vi "SafeMoving.vi"() -> ()   [LabVIEW 2016]
uses:
  Control/SafeControl.ctl
  Control/SafeMoveControl.ctl
  Other Models/2010/Motion/EnableSingle.vi
  Other Models/2010/Motion/DisableSingle.vi
  C:/Users/TTUHEP/Documents/LabVIEW/Other Models/2010/Bin/Aerotech.A3200.dll
  Other Models/2010/Bin/Aerotech.A3200.dll
panel:
  out "Velocity U":dbl
  out "Position U":dbl
  out "Program Position U":dbl
  in  "HOME U":bool
  out "U":string
  out "U":bool
  in  "Enable U":bool
  in  "Axis":enum16{"Z", "Y", "X"}(ring)
  in  "Axis2":string
  in  "Stop3":bool caption="Pause/resume"
  in  "Stop1":bool caption="Pause/resume"
  in  "Move down 2":bool caption="Move"
  in  "Move up 2":bool caption="Move"
  in  "Tab Control":enum32{"Free", "Steps", "Total"}(tab)
  in  "Speed(µm)":dbl=500.0
  in  "Dis/Step(µm)":dbl=5.0
  in  "Step":i32=1
  in  "Dis/step(µm)":dbl=5.0
  in  "Speed(µm/s)":dbl=500.0
  in  "Speed(µm/s) 2":dbl=500.0
  in  "Total Distance(µm)":dbl=5.0
  in  "Dis/step(µm) 2":dbl=1.0
  in  "Pause":bool caption="Pause/resume"
  in  "Resume":bool caption="Pause/resume"
  in  "Move down":bool caption="Move"
  in  "Move up":bool caption="Move"
  out "Boolean":bool
  out "Velocity Z":dbl
  out "Position Z":dbl
  out "Program Position Z":dbl
  out "Velocity Y":dbl
  out "Position Y":dbl
  out "Program Position Y":dbl
  out "Program Position X":dbl
  out "Position X":dbl
  out "Velocity X":dbl format="%#.5g"
  in  "Excute":bool
  in  "HOME Z":bool
  in  "HOME Y":bool
  in  "HOME X":bool
  out "Y":string
  out "Z":string
  out "X":string caption="Status"
  in  "Exit":bool
  out "Z":bool
  out "Y":bool
  out "X":bool
  in  "Enable Z":bool
  in  "Enable Y":bool
  in  "Enable X":bool
  in  "Command":string
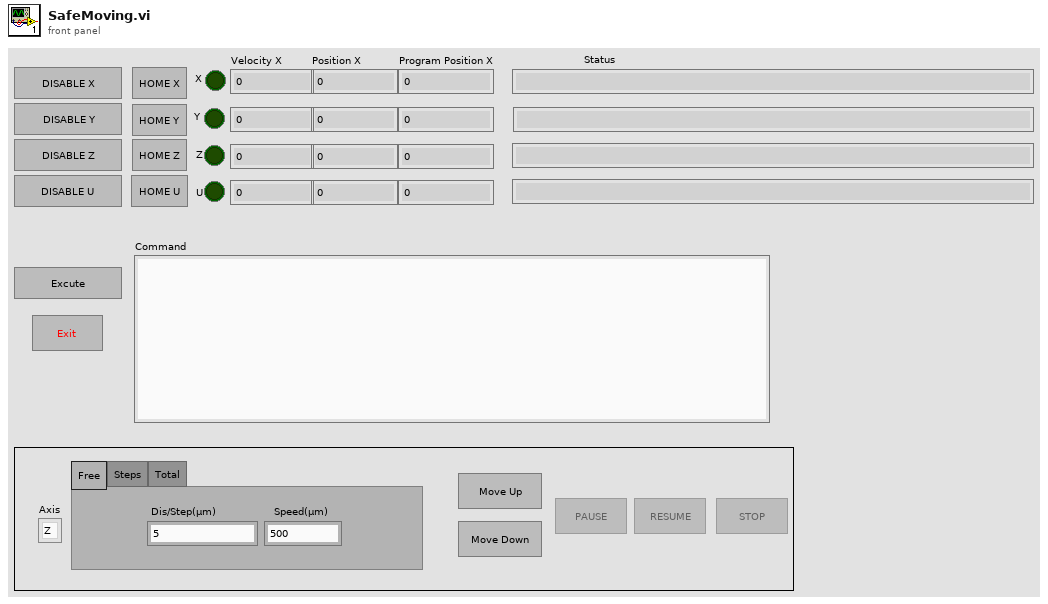
[diagram p1: front panel]
types:
  T1 = typedef "SafeMoveControl.ctl" = enum16{"Idle", "Pause", "Run2", "Run1"}
  T2 = typedef "SafeControl.ctl" = enum16{"Idle", "Abort", "Initialize", "BeforeExcute"}
  T3 = cluster{"X":bool, "Y":bool, "Z":bool, "X":string, "Y":string, "Z":string, "U":bool, "U":string}
  T4 = enum8{"Enabled", "Disabled", "Disabled and Grayed Out"}
  T5 = typedef "ControllerDiagPacket.ctl" = cluster{"Number of Diag Packets":i32, "Axes":T6[], "error":errorcluster}
  T6 = typedef "AxisDiagPacket.ctl" = cluster{"Axis Name":string, "Analog Input 0":dbl, "Analog Input 1":dbl, "Axis Fault (num)":i32, "Axis Fault (str)":string, "Axis Fault (bits)":cluster{"AmplifierFault":bool, "AmplifierTemperatureFault":bool, "CcwEndOfTravelLimitFault":bool, "CcwSoftwareLimitFault":bool, "CommunicationLostFault":bool, "CwEndOfTravelLimitFault":bool, "CwSoftwareLimitFault":bool, "EmergencyStopFault":bool, "EncoderFault":bool, "ExternalFault":bool, "FeedbackScalingFault":bool, "GantryMisalignFault ":bool, "HallSensorFault":bool, "InPositionTimeoutFault":bool, "InternalFault":bool, "MarkerSearchFault":bool, "MaxVelocityCommandFault":bool, "MissedInterruptFault":bool, "MotorTemperatureFault":bool, "None":bool, "OverCurrentFault":bool, "PositionErrorFault":bool, "PositionFeedbackFault":bool, "PowerSupplyFault":bool, "ProbeInputFault":bool, "SafeZoneFault":bool, "VelocityErrorFault":bool, "VelocityFeedbackFault":bool, "VoltageClampFault":bool}, "Axis Status (num)":i32, "Axis Status (str)":string, "Axis Status (bits)":cluster{"BacklashActive":bool, "CalibrationEnabled1D":bool, "CalibrationEnabled2D":bool, "CommandValid":bool, "DriveAbortPending":bool, "DrivePending":bool, "Enabling":bool, "GainMappingEnabled":bool, "GantryAligned":bool, "GantryRealigning":bool, "Homed":bool, "Homing":bool, "IFOVEnabled":bool, "JogGenerating":bool, "Jogging":bool, "JoystickControl":bool, "MasterSlaveControl":bool, "MotionBlocked":bool, "MotionClamped":bool, "MoveDone":bool, "None":bool, "NotVirtual":bool, "Profiling":bool, "Stability0":bool, "Stability1":bool, "TrajectoryFiltering":bool, "WaitDone":bool}, "Current Command":sgl, "Current Error":sgl, "Current Feedback":sgl, "Digital Inputs":i32, "Digital Outputs":i32, "Drive Status":i32, "Drive Status (str)":string, "Drive Status (bits)":cluster{"AccelerationPhase":bool, "AutofocusActive":bool, "BrakeOutput":bool, "CcwEndOfTravelLimitInput":bool, "CosineEncoderError":bool, "CurrentClamp":bool, "CwEndOfTravelLimitInput":bool, "DecelerationPhase":bool, "DualLoopActive":bool, "EmergencyStopInput":bool, "Enabled":bool, "EncoderClipping":bool, "GalvoCalibrationEnabled":bool, "GalvoPowerCorrection":bool, "HallAInput":bool, "HallBInput":bool, "HallCInput":bool, "HighResolutionMode":bool, "HomeLimitInput":bool, "InPosition":bool, "InPosition2":bool, "MarkerInput":bool, "MarkerLatch":bool, "MoveActive":bool, "NoMotorSupply":bool, "None":bool, "PowerLimiting":bool, "ProgrammingFlash":bool, "ProgrammingMXH":bool, "PSOHaltLatch":bool, "ServoControl":bool, "SineEncoderError":bool}, "Position Feedback Auxiliary":dbl, "Position Command":dbl, "Position Error":dbl, "Position Feedback":dbl, "Program Position Command":dbl, "Program Position Error":dbl, "Program Position Feedback":dbl, "Velocity Command":dbl, "Velocity Error":dbl, "Velocity Feedback":dbl}
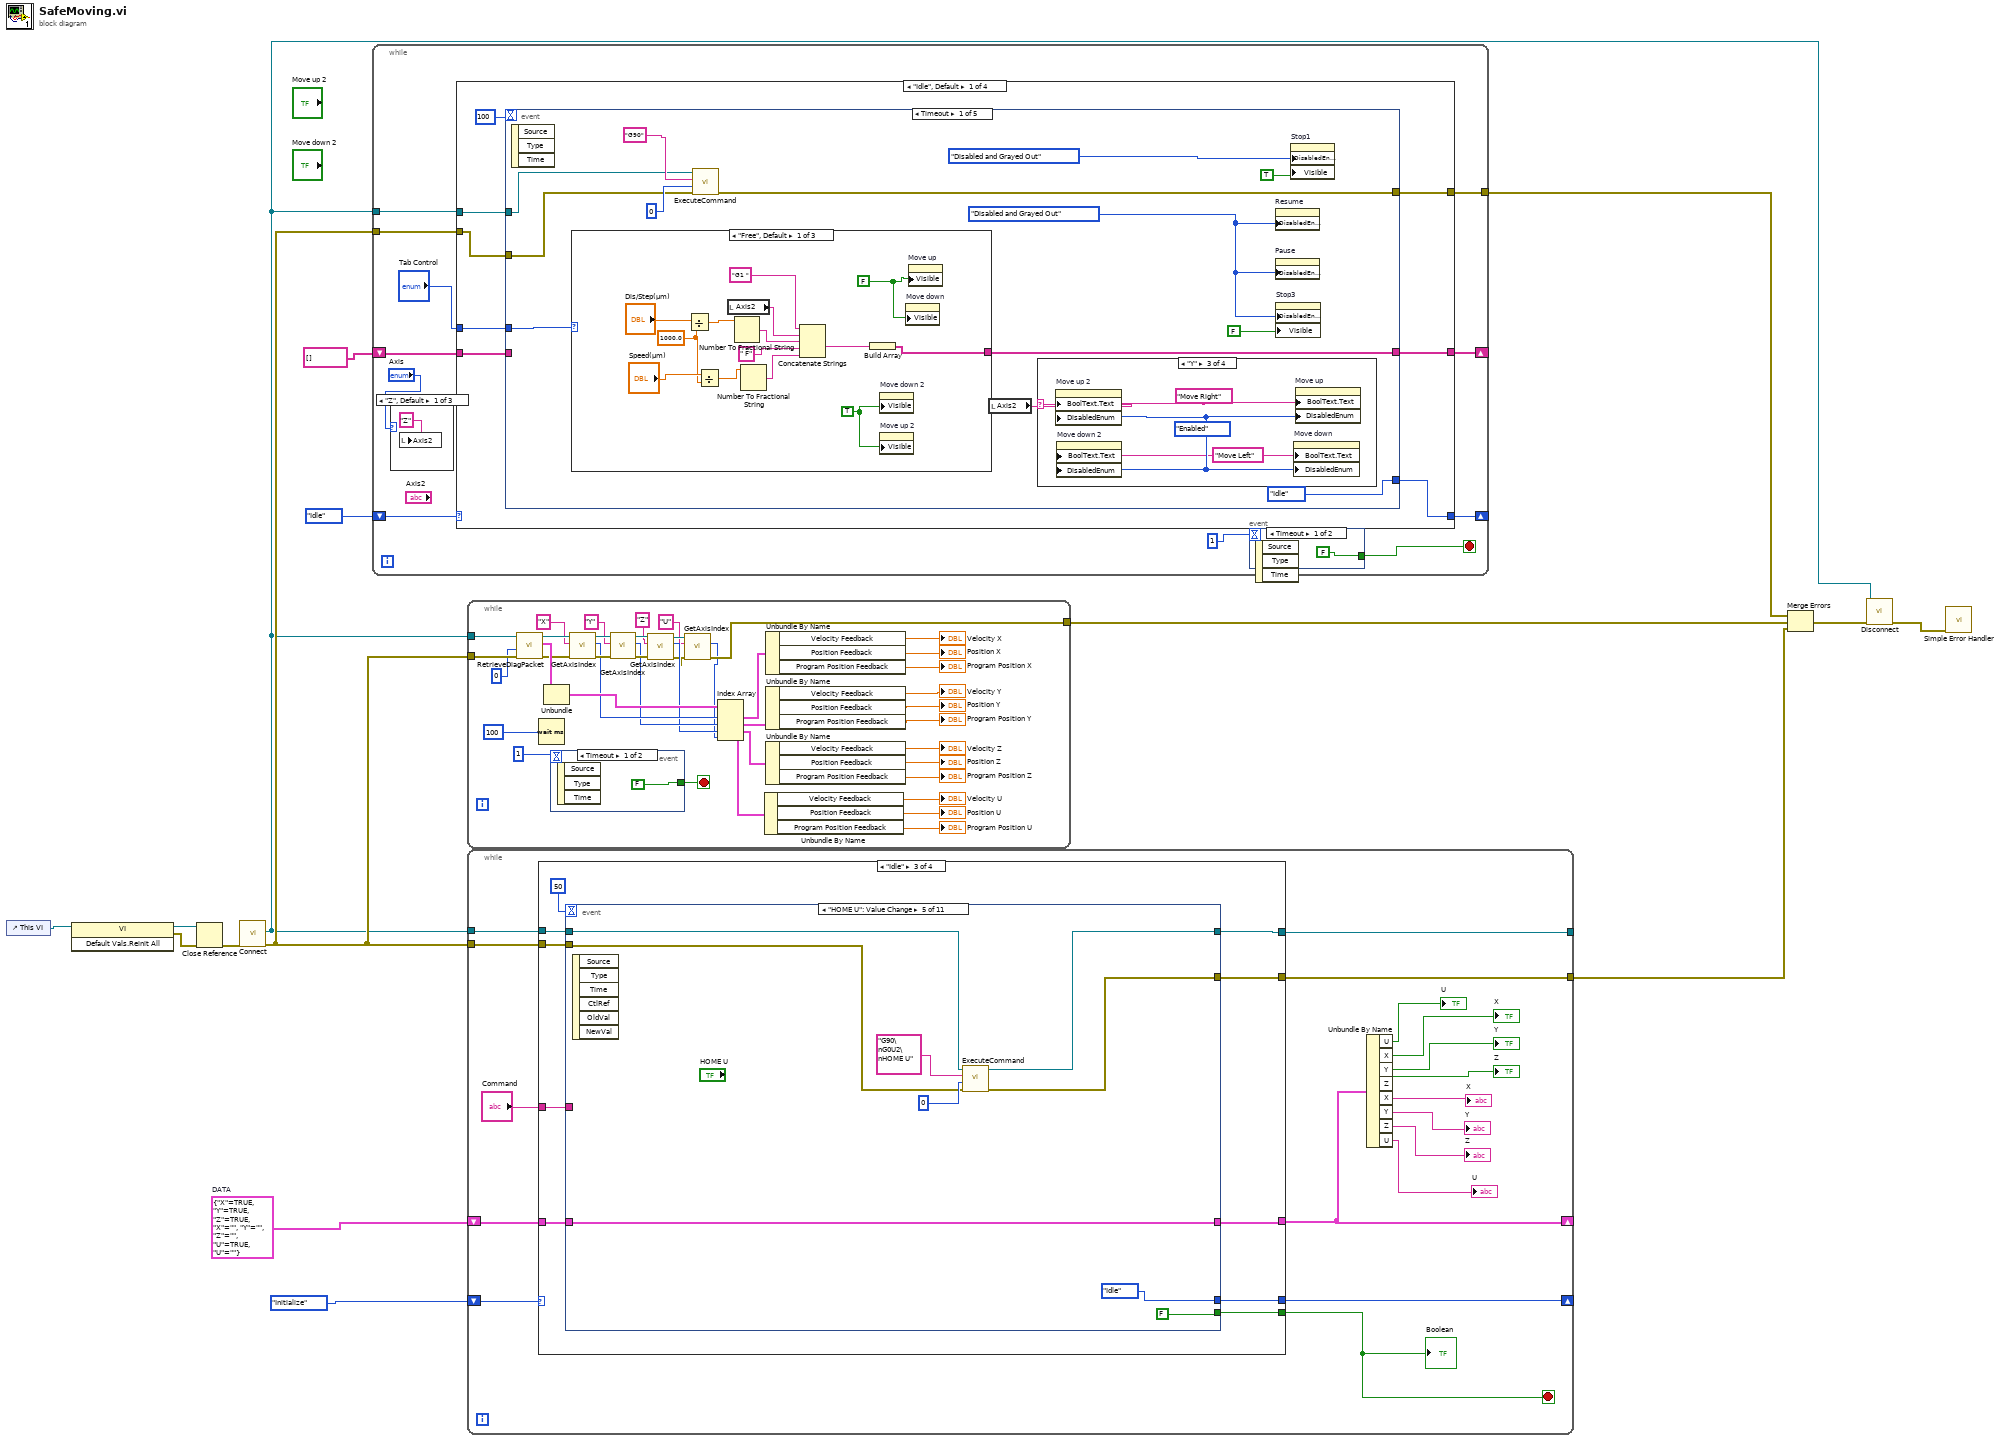
[diagram p0: block diagram]
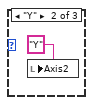
[diagram p2: hidden frame]
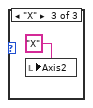
[diagram p3: hidden frame]
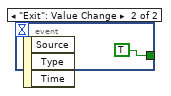
[diagram p4: hidden frame]
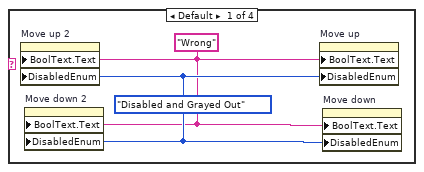
[diagram p5: hidden frame]
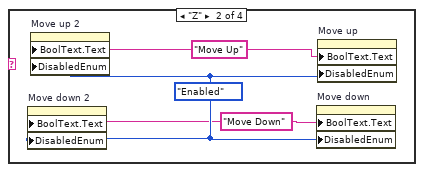
[diagram p6: hidden frame]
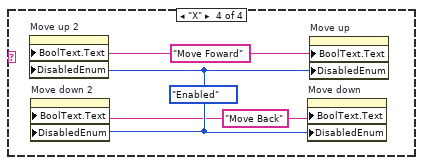
[diagram p7: hidden frame]
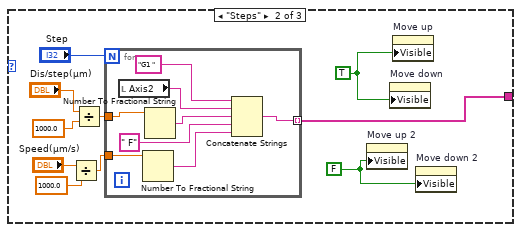
[diagram p8: hidden frame]
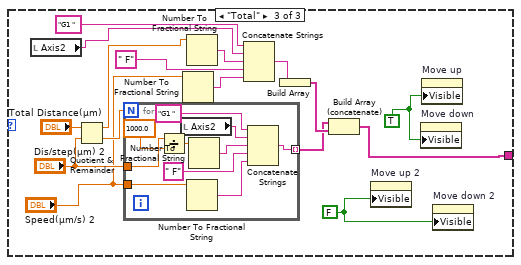
[diagram p9: hidden frame]
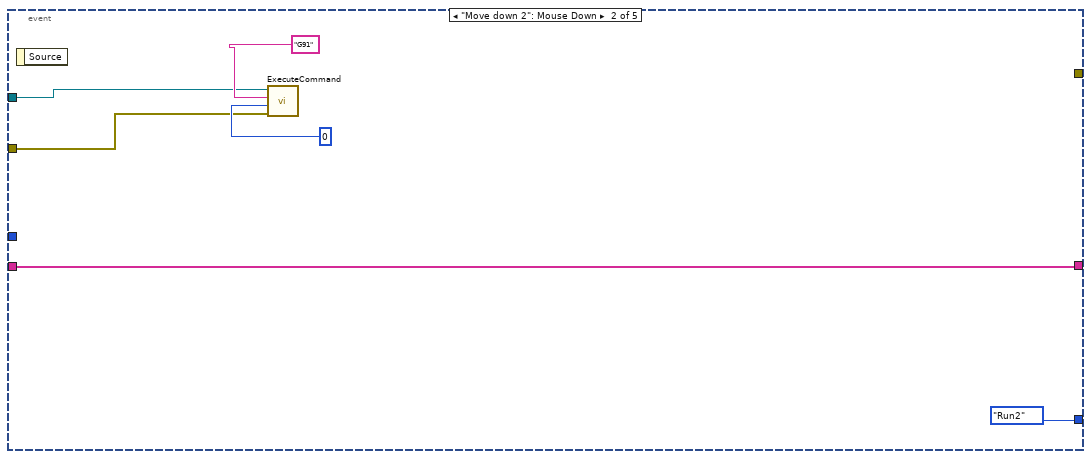
[diagram p10: hidden frame]
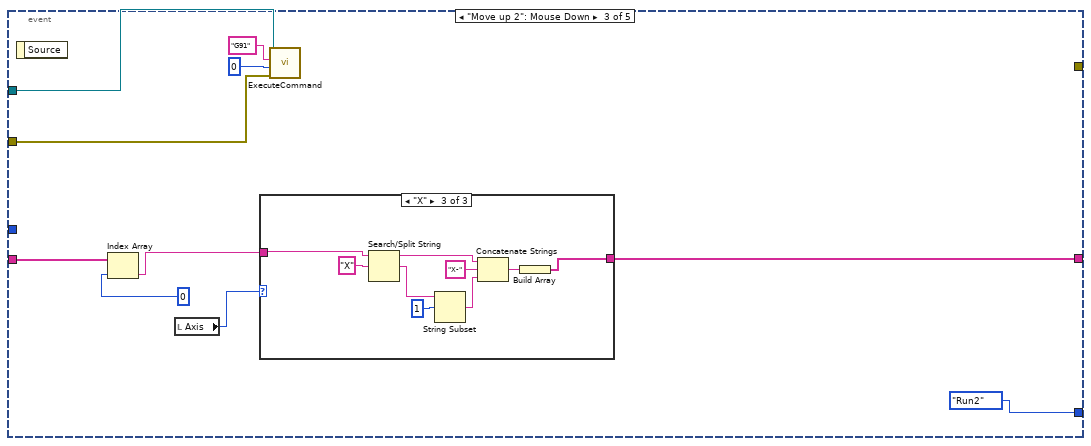
[diagram p11: hidden frame]
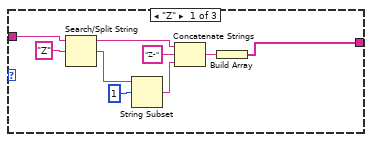
[diagram p12: hidden frame]
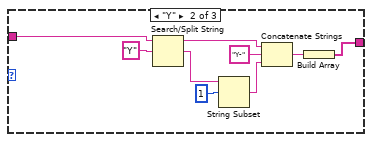
[diagram p13: hidden frame]
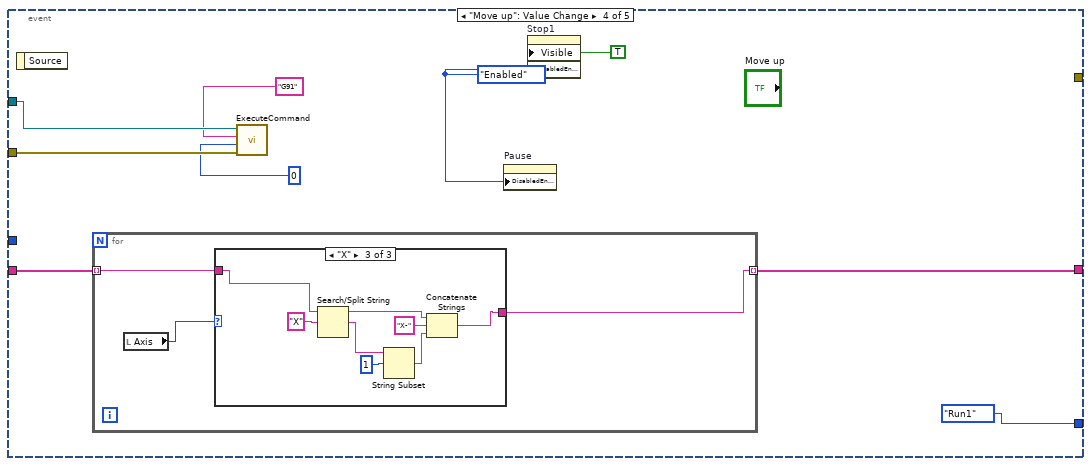
[diagram p14: hidden frame]
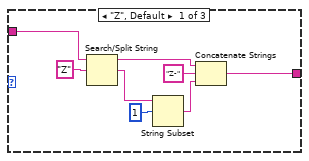
[diagram p15: hidden frame]
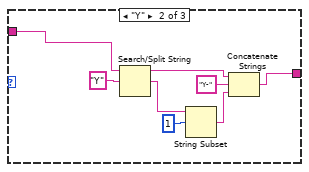
[diagram p16: hidden frame]
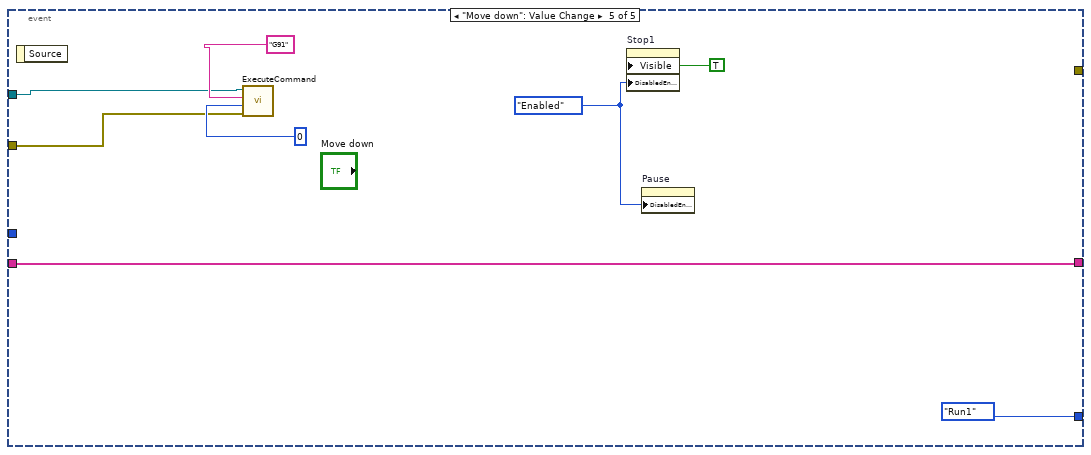
[diagram p17: hidden frame]
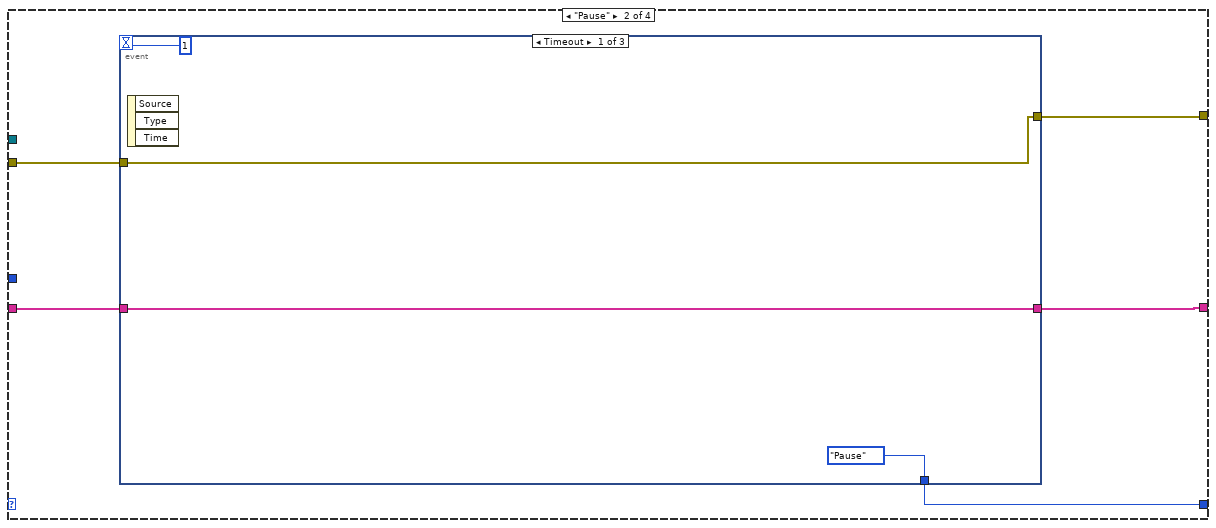
[diagram p18: hidden frame]
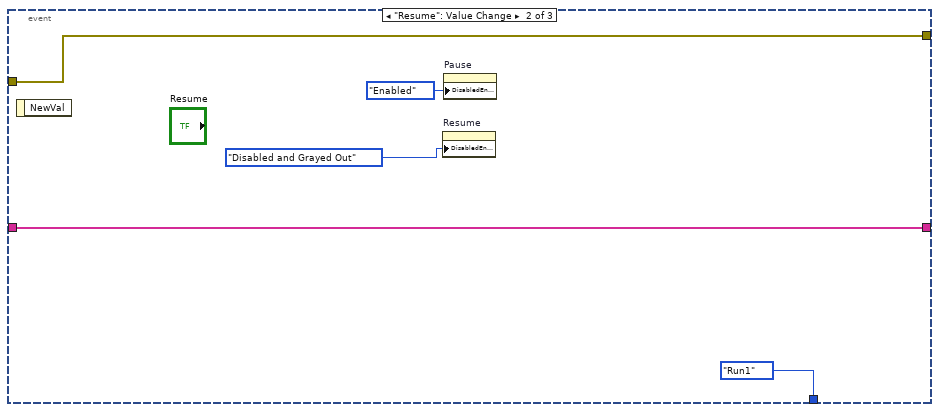
[diagram p19: hidden frame]
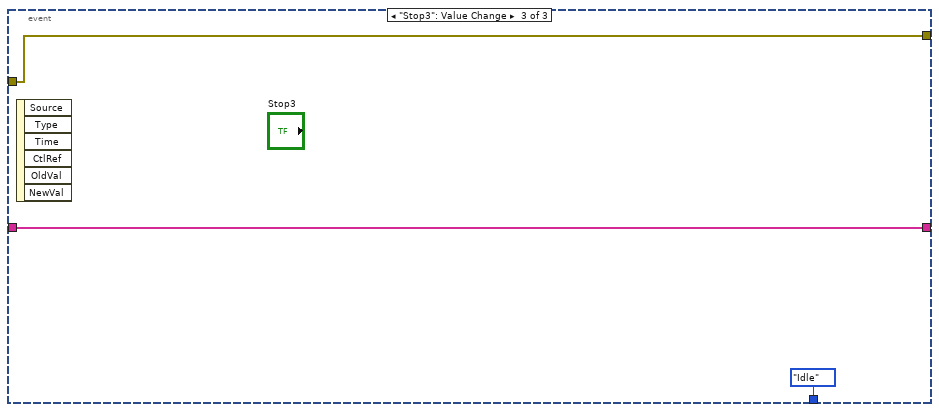
[diagram p20: hidden frame]
diagram:
  w15 = T3 {"X"=TRUE, "Y"=TRUE, "Z"=TRUE, "X"="", "Y"="", "Z"="", "U"=TRUE, "U"=""}  # DATA
  n1 = control-ref of="This VI"() -> (w13:refnum<vi>)
  n2 = invoke class="VI" method="Default Vals.Reinit All"(reference=w13) -> (reference out=w12:refnum<vi>, error out=w11:errorcluster)  [unwired: 2 in, 1 out]
  n3 = Close Reference(reference=w12, error in (no error)=w11) -> (error out=w10:errorcluster)
  n4 = call "Connect.vi"("error in (no error)"=w10) -> ("error out"=w3:errorcluster, "controller"=w2:refnum<k24>)  [unwired: 9 in]
  n5 = while {
    tunnel: w2 -> [w24]
    tunnel: w3 -> [w23]
    shift-right: [w25] -> _
    shift-left: SafeMoveControl."Idle" -> [w26]
    shift-right: [w21] -> _
    shift-left: string[] [] -> [w20]
    tunnel: [w17] -> w1
    stop <- w18 stop-if-true
    n6 = case shown="\"Z\", Default" "Axis" {
      frame "Z", Default {
        n7 = local write "Axis2"("Z") -> ()
      }
      frame "Y" {
        n8 = local write "Axis2"("Y") -> ()
      }
      frame "X" {
        n9 = local write "Axis2"("X") -> ()
      }
    }
    n10 = case shown="\"Idle\", Default" w26 {
      tunnel: [w39 w212 w230 w252] -> w25
      tunnel: w24 -> [w34 _ w229 w250]
      tunnel: w23 -> [w33 w211 w228 w251]
      tunnel: "Tab Control" -> [w38 _ _ _]
      tunnel: [w37 w213 w227 w248] -> w21
      tunnel: w20 -> [w36 w214 w231 w249]
      tunnel: [w32 w210 w226 w247] -> w17
      frame "Idle", Default {
        n11 = event shown="[0] Timeout" {
          selector: _ -> [_ _ _ _ _]
          dyn-events: _ -> [_ _ _ _ _]
          timeout: 100 -> [_ _ _ _ _]
          tunnel: [enum16{"Idle"}."Idle" SafeMoveControl."Run2" SafeMoveControl."Run2" SafeMoveControl."Run1" SafeMoveControl."Run1"] -> w39
          tunnel: w38 -> [w51 _ _ _ _]
          tunnel: [w50 w126 w133 w171 w207] -> w37
          tunnel: w36 -> [_ w126 w136 w172 w207]
          tunnel: w34 -> [w47 w123 w130 w170 w204]
          tunnel: w33 -> [w46 w122 w129 w169 w203]
          tunnel: [w45 _ _ _ _] -> w32
          event Timeout {
            w42 = T4."Disabled and Grayed Out" ("Disabled")
            n12 = event-data() -> ()  [unwired: 1 in, 3 out]
            n13 = case shown="\"Free\", Default" w51 {
              tunnel: [w71 w86 w100] -> w50
              frame "Free", Default {
                w66 = 1000.0
                w76 = TRUE
                w77 = FALSE
                n14 = Divide(x="Dis/Step(µm)", y=w66) -> (x/y=w69:dbl)
                n15 = Divide(x="Speed(µm)", y=w66) -> (x/y=w68:dbl)
                n16 = local read "Axis2"() -> (w64:string)
                n17 = Number To Fractional String(number=w69) -> (F-format string=w75:string)  [unwired: 3 in]
                n18 = Number To Fractional String(number=w68) -> (F-format string=w73:string)  [unwired: 3 in]
                n19 = Concatenate Strings("G1 ", w64, w75, " F", w73) -> (w72:string)
                n20 = Build Array(w72) -> (w71:string[])
                n21 = property on="Move down 2" class="Bool (strict)"("Visible"=w76) -> ()  [unwired: 2 in, 2 out]
                n22 = property on="Move up 2" class="Bool (strict)"("Visible"=w76) -> ()  [unwired: 2 in, 2 out]
                n23 = property on="Move down" class="Bool"("Visible"=w77) -> ()  [unwired: 2 in, 2 out]
                n24 = property on="Move up" class="Bool"("Visible"=w77) -> ()  [unwired: 2 in, 2 out]
              }
              frame "Steps" {
                w81 = FALSE
                w82 = TRUE
                n25 = Divide(x="Speed(µm/s)", y=1000.0) -> (x/y=w83:dbl)
                n26 = Divide(x="Dis/step(µm)", y=1000.0) -> (x/y=w78:dbl)
                n27 = for {
                  N: "Step" -> [_]
                  tunnel: w83 -> [w95]
                  tunnel: [w91] -> w86 mode=indexing
                  tunnel: w78 -> [w90]
                  n28 = local read "Axis2"() -> (w88:string)
                  n29 = Number To Fractional String(number=w95) -> (F-format string=w92:string)  [unwired: 3 in]
                  n30 = Number To Fractional String(number=w90) -> (F-format string=w94:string)  [unwired: 3 in]
                  n31 = Concatenate Strings("G1 ", w88, w94, " F", w92) -> (w91:string)
                }
                n32 = property on="Move up 2" class="Bool (strict)"("Visible"=w81) -> ()  [unwired: 2 in, 2 out]
                n33 = property on="Move down" class="Bool"("Visible"=w82) -> ()  [unwired: 2 in, 2 out]
                n34 = property on="Move up" class="Bool"("Visible"=w82) -> ()  [unwired: 2 in, 2 out]
                n35 = property on="Move down 2" class="Bool (strict)"("Visible"=w81) -> ()  [unwired: 2 in, 2 out]
              }
              frame "Total" {
                w110 = FALSE
                w111 = TRUE
                n36 = local read "Axis2"() -> (w96:string)
                n37 = Quotient & Remainder(x="Total Distance(µm)", y="Dis/step(µm) 2") -> (x-y*floor(x/y)=w102:dbl, floor(x/y)=w108:dbl)
                n38 = for {
                  N: w108 -> [_]
                  tunnel: "Speed(µm/s) 2" -> [w119]
                  tunnel: "Dis/step(µm) 2" -> [w115]
                  tunnel: [w117] -> w98 mode=indexing
                  n39 = Divide(x=w115, y=1000.0) -> (x/y=w116:dbl)
                  n40 = local read "Axis2"() -> (w112:string)
                  n41 = Number To Fractional String(number=w119) -> (F-format string=w118:string)  [unwired: 3 in]
                  n42 = Number To Fractional String(number=w116) -> (F-format string=w121:string)  [unwired: 3 in]
                  n43 = Concatenate Strings("G1 ", w112, w121, " F", w118) -> (w117:string)
                }
                n44 = Number To Fractional String(number="Speed(µm/s) 2") -> (F-format string=w104:string)  [unwired: 3 in]
                n45 = Number To Fractional String(number=w102) -> (F-format string=w103:string)  [unwired: 3 in]
                n46 = Concatenate Strings("G1 ", w96, w103, " F", w104) -> (w106:string)
                n47 = Build Array(w106) -> (w99:string[])
                n48 = Build Array (concatenate)(w98, w99) -> (w100:string[])
                n49 = property on="Move up 2" class="Bool (strict)"("Visible"=w110) -> ()  [unwired: 2 in, 2 out]
                n50 = property on="Move down" class="Bool"("Visible"=w111) -> ()  [unwired: 2 in, 2 out]
                n51 = property on="Move up" class="Bool"("Visible"=w111) -> ()  [unwired: 2 in, 2 out]
                n52 = property on="Move down 2" class="Bool (strict)"("Visible"=w110) -> ()  [unwired: 2 in, 2 out]
              }
            }
            n53 = call "ExecuteCommand.vi"("error in (no error)"=w46, "taskId"=0, "Command Code"="G90", "controller in"=w47) -> ("error out"=w45:errorcluster)  [unwired: 5 in, 2 out]
            n54 = local read "Axis2"() -> (w40:string)
            n55 = case shown="\"Y\"" w40 {
              frame Default {
                w54 = T4."Disabled and Grayed Out" ("Disabled")
                w53 = "Wrong"
                n56 = property on="Move up 2" class="Bool (strict)"("BoolText.Text"=w53, "DisabledEnum"=w54) -> ()  [unwired: 2 in, 2 out]
                n57 = property on="Move down 2" class="Bool (strict)"("BoolText.Text"=w53, "DisabledEnum"=w54) -> ()  [unwired: 2 in, 2 out]
                n58 = property on="Move up" class="Bool"("BoolText.Text"=w53, "DisabledEnum"=w54) -> ()  [unwired: 2 in, 2 out]
                n59 = property on="Move down" class="Bool"("BoolText.Text"=w53, "DisabledEnum"=w54) -> ()  [unwired: 2 in, 2 out]
              }
              frame "Z" {
                w55 = "Move Down"
                w57 = T4."Enabled" ("Disabled")
                w56 = "Move Up"
                n60 = property on="Move down 2" class="Bool (strict)"("BoolText.Text"=w55, "DisabledEnum"=w57) -> ()  [unwired: 2 in, 2 out]
                n61 = property on="Move up 2" class="Bool (strict)"("BoolText.Text"=w56, "DisabledEnum"=w57) -> ()  [unwired: 2 in, 2 out]
                n62 = property on="Move down" class="Bool"("BoolText.Text"=w55, "DisabledEnum"=w57) -> ()  [unwired: 2 in, 2 out]
                n63 = property on="Move up" class="Bool"("BoolText.Text"=w56, "DisabledEnum"=w57) -> ()  [unwired: 2 in, 2 out]
              }
              frame "Y" {
                w58 = "Move Left"
                w60 = T4."Enabled" ("Disabled")
                w59 = "Move Right"
                n64 = property on="Move up 2" class="Bool (strict)"("BoolText.Text"=w59, "DisabledEnum"=w60) -> ()  [unwired: 2 in, 2 out]
                n65 = property on="Move down 2" class="Bool (strict)"("BoolText.Text"=w58, "DisabledEnum"=w60) -> ()  [unwired: 2 in, 2 out]
                n66 = property on="Move down" class="Bool"("BoolText.Text"=w58, "DisabledEnum"=w60) -> ()  [unwired: 2 in, 2 out]
                n67 = property on="Move up" class="Bool"("BoolText.Text"=w59, "DisabledEnum"=w60) -> ()  [unwired: 2 in, 2 out]
              }
              frame "X" {
                w61 = "Move Back"
                w63 = T4."Enabled" ("Disabled")
                w62 = "Move Foward"
                n68 = property on="Move up 2" class="Bool (strict)"("BoolText.Text"=w62, "DisabledEnum"=w63) -> ()  [unwired: 2 in, 2 out]
                n69 = property on="Move down 2" class="Bool (strict)"("BoolText.Text"=w61, "DisabledEnum"=w63) -> ()  [unwired: 2 in, 2 out]
                n70 = property on="Move down" class="Bool"("BoolText.Text"=w61, "DisabledEnum"=w63) -> ()  [unwired: 2 in, 2 out]
                n71 = property on="Move up" class="Bool"("BoolText.Text"=w62, "DisabledEnum"=w63) -> ()  [unwired: 2 in, 2 out]
              }
            }
            n72 = property on="Resume" class="Bool"("DisabledEnum"=w42) -> ()  [unwired: 2 in, 2 out]
            n73 = property on="Pause" class="Bool"("DisabledEnum"=w42) -> ()  [unwired: 2 in, 2 out]
            n74 = property on="Stop3" class="Bool"("DisabledEnum"=w42, "Visible"=FALSE) -> ()  [unwired: 2 in, 2 out]
            n75 = property on="Stop1" class="Bool"("DisabledEnum"=T4."Disabled and Grayed Out" ("Disabled"), "Visible"=TRUE) -> ()  [unwired: 2 in, 2 out]
          }
          event "Move down 2": Mouse Down {
            n76 = event-data() -> ()  [unwired: 1 in, 1 out]
            n77 = call "ExecuteCommand.vi"("error in (no error)"=w122, "taskId"=0, "Command Code"="G91", "controller in"=w123) -> ()  [unwired: 5 in, 3 out]
          }
          event "Move up 2": Mouse Down {
            n78 = event-data() -> ()  [unwired: 1 in, 1 out]
            n79 = Index Array(array=w136, index=0) -> (element=w134:string)
            n80 = local read "Axis"() -> (w128:enum16{"Z", "Y", "X"})
            n81 = case shown="\"X\"" w128 {
              tunnel: w134 -> [w140 w148 w157]
              tunnel: [w138 w147 w156] -> w133
              frame "Z" {
                n82 = Search/Split String(string=w140, search string/char (-)="Z") -> (substring before match=w143:string, match + rest of string=w145:string)  [unwired: 1 in, 1 out]
                n83 = String Subset(string=w145, offset (0)=1) -> (substring=w141:string)  [unwired: 1 in]
                n84 = Concatenate Strings(w143, "Z-", w141) -> (w139:string)
                n85 = Build Array(w139) -> (w138:string[])
              }
              frame "Y" {
                n86 = Search/Split String(string=w148, search string/char (-)="Y") -> (substring before match=w152:string, match + rest of string=w154:string)  [unwired: 1 in, 1 out]
                n87 = String Subset(string=w154, offset (0)=1) -> (substring=w150:string)  [unwired: 1 in]
                n88 = Concatenate Strings(w152, "Y-", w150) -> (w149:string)
                n89 = Build Array(w149) -> (w147:string[])
              }
              frame "X" {
                n90 = Search/Split String(string=w157, search string/char (-)="X") -> (substring before match=w161:string, match + rest of string=w159:string)  [unwired: 1 in, 1 out]
                n91 = String Subset(string=w159, offset (0)=1) -> (substring=w163:string)  [unwired: 1 in]
                n92 = Concatenate Strings(w161, "X-", w163) -> (w164:string)
                n93 = Build Array(w164) -> (w156:string[])
              }
            }
            n94 = call "ExecuteCommand.vi"("error in (no error)"=w129, "taskId"=0, "Command Code"="G91", "controller in"=w130) -> ()  [unwired: 5 in, 3 out]
          }
          event "Move up": Value Change {
            w165 = T4."Enabled" ("Disabled")
            n95 = event-data() -> ()  [unwired: 1 in, 1 out]
            n96 = for {
              tunnel: w172 -> [w176] mode=indexing
              tunnel: [w175] -> w171 mode=indexing
              n97 = local read "Axis"() -> (w174:enum16{"Z", "Y", "X"})
              n98 = case shown="\"X\"" w174 {
                tunnel: w176 -> [w184 w186 w193]
                tunnel: [w177 w185 w194] -> w175
                frame "Z", Default {
                  n99 = Search/Split String(string=w184, search string/char (-)="Z") -> (substring before match=w180:string, match + rest of string=w182:string)  [unwired: 1 in, 1 out]
                  n100 = String Subset(string=w182, offset (0)=1) -> (substring=w178:string)  [unwired: 1 in]
                  n101 = Concatenate Strings(w180, "Z-", w178) -> (w177:string)
                }
                frame "Y" {
                  n102 = Search/Split String(string=w186, search string/char (-)="Y") -> (substring before match=w190:string, match + rest of string=w188:string)  [unwired: 1 in, 1 out]
                  n103 = String Subset(string=w188, offset (0)=1) -> (substring=w192:string)  [unwired: 1 in]
                  n104 = Concatenate Strings(w190, "Y-", w192) -> (w185:string)
                }
                frame "X" {
                  n105 = Search/Split String(string=w193, search string/char (-)="X") -> (substring before match=w197:string, match + rest of string=w199:string)  [unwired: 1 in, 1 out]
                  n106 = String Subset(string=w199, offset (0)=1) -> (substring=w195:string)  [unwired: 1 in]
                  n107 = Concatenate Strings(w197, "X-", w195) -> (w194:string)
                }
              }
            }
            n108 = call "ExecuteCommand.vi"("error in (no error)"=w169, "taskId"=0, "Command Code"="G91", "controller in"=w170) -> ()  [unwired: 5 in, 3 out]
            n109 = property on="Pause" class="Bool"("DisabledEnum"=w165) -> ()  [unwired: 2 in, 2 out]
            n110 = property on="Stop1" class="Bool"("Visible"=TRUE, "DisabledEnum"=w165) -> ()  [unwired: 2 in, 2 out]
          }
          event "Move down": Value Change {
            w202 = T4."Enabled" ("Disabled")
            n111 = event-data() -> ()  [unwired: 1 in, 1 out]
            n112 = call "ExecuteCommand.vi"("error in (no error)"=w203, "taskId"=0, "Command Code"="G91", "controller in"=w204) -> ()  [unwired: 5 in, 3 out]
            n113 = property on="Stop1" class="Bool"("Visible"=TRUE, "DisabledEnum"=w202) -> ()  [unwired: 2 in, 2 out]
            n114 = property on="Pause" class="Bool"("DisabledEnum"=w202) -> ()  [unwired: 2 in, 2 out]
          }
        }
      }
      frame "Pause" {
        n115 = event shown="[0] Timeout" {
          selector: _ -> [_ _ _]
          dyn-events: _ -> [_ _ _]
          timeout: 1 -> [_ _ _]
          tunnel: w214 -> [w217 w222 w224]
          tunnel: [w217 w222 w224] -> w213
          tunnel: [SafeMoveControl."Pause" SafeMoveControl."Run1" SafeMoveControl."Idle"] -> w212
          tunnel: w211 -> [w215 w218 w225]
          tunnel: [w215 w218 w225] -> w210
          event Timeout {
            n116 = event-data() -> ()  [unwired: 1 in, 3 out]
          }
          event "Resume": Value Change {
            n117 = event-data() -> ()  [unwired: 1 in, 1 out]
            n118 = property on="Resume" class="Bool"("DisabledEnum"=T4."Disabled and Grayed Out" ("Disabled")) -> ()  [unwired: 2 in, 2 out]
            n119 = property on="Pause" class="Bool"("DisabledEnum"=T4."Enabled" ("Disabled")) -> ()  [unwired: 2 in, 2 out]
          }
          event "Stop3": Value Change {
            n120 = event-data() -> ()  [unwired: 1 in, 6 out]
          }
        }
      }
      frame "Run2" {
        n121 = event shown="[1] \"Move down 2\": Mouse Up" {
          selector: _ -> [_ _ _]
          dyn-events: _ -> [_ _ _]
          timeout: 10 -> [_ _ _]
          tunnel: w231 -> [w235 w242 w245]
          tunnel: [SafeMoveControl."Run2" SafeMoveControl."Idle" SafeMoveControl."Idle"] -> w230
          tunnel: w229 -> [w239 _ _]
          tunnel: w228 -> [w238 w241 w244]
          tunnel: [w235 w242 w245] -> w227
          tunnel: [w233 w241 w244] -> w226
          event Timeout {
            n122 = event-data() -> ()  [unwired: 1 in, 3 out]
            n123 = Index Array(array=w235, index=0) -> (element=w237:string)
            n124 = call "ExecuteCommand.vi"("error in (no error)"=w238, "taskId"=0, "Command Code"=w237, "controller in"=w239) -> ("error out"=w233:errorcluster)  [unwired: 5 in, 2 out]
          }
          event "Move down 2": Mouse Up {
            n125 = event-data() -> ()  [unwired: 1 in, 1 out]
          }
          event "Move up 2": Mouse Up {
            n126 = event-data() -> ()  [unwired: 1 in, 1 out]
          }
        }
      }
      frame "Run1" {
        n127 = event shown="[0] Timeout" {
          selector: _ -> [_ _ _]
          dyn-events: _ -> [_ _ _]
          timeout: 10 -> [_ _ _]
          tunnel: [w255 SafeMoveControl."Pause" SafeMoveControl."Idle"] -> w252
          tunnel: w251 -> [w261 w282 w289]
          tunnel: w250 -> [w262 _ _]
          tunnel: w249 -> [w259 w285 w288]
          tunnel: [w260 w285 w288] -> w248
          tunnel: [w254 w282 w289] -> w247
          event Timeout {
            n128 = event-data() -> ()  [unwired: 1 in, 1 out]
            n129 = Array Size(array=w259) -> (size(s)=w258:i32)
            n130 = Greater Or Equal?(x=w258, y=1) -> (x >= y?=w256:bool)
            n131 = case shown="True" w256 {
              tunnel: w262 -> [_ w277]
              tunnel: w261 -> [w263 w276]
              tunnel: [w265 w268] -> w260
              tunnel: w259 -> [w265 w270]
              tunnel: [SafeMoveControl."Idle" SafeMoveControl."Run1"] -> w255
              tunnel: [w263 w266] -> w254
              frame False {
              }
              frame True {
                n132 = Delete From Array(array=w270, length=1, index=0) -> (deleted portion=w267:string[], array with subset deleted=w268:string[])
                n133 = Index Array(array=w267, index=0) -> (element=w273:string)
                n134 = call "ExecuteCommand.vi"("error in (no error)"=w276, "taskId"=0, "Command Code"=w273, "controller in"=w277) -> ("error out"=w266:errorcluster)  [unwired: 5 in, 2 out]
              }
            }
          }
          event "Pause": Value Change {
            n135 = event-data() -> ()  [unwired: 1 in, 1 out]
            n136 = property on="Resume" class="Bool"("DisabledEnum"=T4."Enabled" ("Disabled")) -> ()  [unwired: 2 in, 2 out]
            n137 = property on="Pause" class="Bool"("DisabledEnum"=T4."Disabled and Grayed Out" ("Disabled")) -> ()  [unwired: 2 in, 2 out]
            n138 = property on="Stop1" class="Bool"("DisabledEnum"=T4."Disabled and Grayed Out" ("Disabled"), "Visible"=FALSE) -> ()  [unwired: 2 in, 2 out]
            n139 = property on="Stop3" class="Bool"("DisabledEnum"=T4."Enabled" ("Disabled"), "Visible"=TRUE) -> ()  [unwired: 2 in, 2 out]
          }
          event "Stop1": Value Change {
            n140 = event-data() -> ()  [unwired: 1 in, 1 out]
          }
        }
      }
    }
    n141 = event shown="[0] Timeout" {
      selector: _ -> [_ _]
      dyn-events: _ -> [_ _]
      timeout: 1 -> [_ _]
      tunnel: [FALSE TRUE] -> w18
      event Timeout {
        n142 = event-data() -> ()  [unwired: 1 in, 3 out]
      }
      event "Exit": Value Change {
        n143 = event-data() -> ()  [unwired: 1 in, 3 out]
      }
    }
  }
  n144 = while {
    tunnel: w2 -> [w317]
    tunnel: w3 -> [w316]
    tunnel: [w295] -> w4
    stop <- w302 stop-if-true
    n145 = call "RetrieveDiagPacket.vi"("error in (no error)"=w316, "axisMask"=0, "Controller In"=w317) -> ("error out"=w329:errorcluster, "ControllerDiagPacket"=w330:T5, "Controller Out"=w328:refnum<k24>)  [unwired: 6 in]
    n146 = Wait (ms)(milliseconds to wait=100) -> ()  [unwired: 1 out]
    n147 = Unbundle(w330) -> ("Axes"=w321:T6[])  [unwired: 2 out]
    n148 = event shown="[0] Timeout" {
      selector: _ -> [_ _]
      dyn-events: _ -> [_ _]
      timeout: 1 -> [_ _]
      tunnel: [FALSE TRUE] -> w302
      event Timeout {
        n149 = event-data() -> ()  [unwired: 1 in, 3 out]
      }
      event "Exit": Value Change {
        n150 = event-data() -> ()  [unwired: 1 in, 3 out]
      }
    }
    n151 = call "GetAxisIndex.vi"("error in (no error)"=w329, "axis name"="X", "controller in"=w328) -> ("error out"=w325:errorcluster, "axis index"=w320:i32, "controller out"=w327:refnum<k24>)  [unwired: 6 in]
    n152 = call "GetAxisIndex.vi"("error in (no error)"=w325, "axis name"="Y", "controller in"=w327) -> ("error out"=w324:errorcluster, "axis index"=w319:i32, "controller out"=w326:refnum<k24>)  [unwired: 6 in]
    n153 = call "GetAxisIndex.vi"("error in (no error)"=w324, "axis name"="Z", "controller in"=w326) -> ("error out"=w297:errorcluster, "axis index"=w318:i32, "controller out"=w298:refnum<k24>)  [unwired: 6 in]
    n154 = call "GetAxisIndex.vi"("error in (no error)"=w297, "axis name"="U", "controller in"=w298) -> ("error out"=w295:errorcluster, "axis index"=w294:i32)  [unwired: 6 in, 1 out]
    n155 = Index Array(array=w321, index #1=w320, index #2=w319, index #3=w318, index #4=w294) -> (element #1=w314:T6, element #2=w312:T6, element #3=w313:T6, element #4=w293:T6)
    n156 = Unbundle By Name(w293) -> ("Velocity Feedback"=→"Velocity U":dbl, "Position Feedback"=→"Position U":dbl, "Program Position Feedback"=→"Program Position U":dbl)
    n157 = Unbundle By Name(w314) -> ("Velocity Feedback"=→"Velocity X":dbl, "Position Feedback"=→"Position X":dbl, "Program Position Feedback"=→"Program Position X":dbl)
    n158 = Unbundle By Name(w312) -> ("Velocity Feedback"=→"Velocity Y":dbl, "Position Feedback"=→"Position Y":dbl, "Program Position Feedback"=→"Program Position Y":dbl)
    n159 = Unbundle By Name(w313) -> ("Velocity Feedback"=→"Velocity Z":dbl, "Position Feedback"=→"Position Z":dbl, "Program Position Feedback"=→"Program Position Z":dbl)
  }
  n160 = while {
    tunnel: w2 -> [w350]
    tunnel: w3 -> [w349]
    shift-right: [w344] -> _
    shift-left: SafeControl."Initialize" -> [w341]
    shift-right: [w343] -> _
    shift-left: w15 -> [w348]
    tunnel: [w342] -> _
    tunnel: [w335] -> w7
    stop <- w336 stop-if-true
    n161 = case shown="\"Idle\"" w341 {
      tunnel: w350 -> [w355 w384 w402 w574]
      tunnel: w349 -> [w351 w383 w403 w571]
      tunnel: w348 -> [w354 w368 w401 w572]
      tunnel: [w354 w367 w395 w572] -> w343
      tunnel: [SafeControl."Idle" SafeControl."Idle" w400 SafeControl."Idle"] -> w344
      tunnel: [w355 w366 w399 w574] -> w342
      tunnel: [FALSE FALSE w397 TRUE] -> w336
      tunnel: "Command" -> [_ _ w396 _]
      tunnel: [w351 w357 w394 w571] -> w335
      frame "BeforeExcute" {
      }
      frame "Initialize" {
        n162 = call "RetrieveDiagPacket.vi"("error in (no error)"=w383, "axisMask"=0, "Controller In"=w384) -> ("error out"=w386:errorcluster, "ControllerDiagPacket"=w387:T5, "Controller Out"=w385:refnum<k24>)  [unwired: 6 in]
        n163 = Unbundle(w387) -> ("Axes"=w375:T6[])  [unwired: 2 out]
        n164 = call "GetAxisIndex.vi"("error in (no error)"=w386, "axis name"="X", "controller in"=w385) -> ("error out"=w380:errorcluster, "axis index"=w374:i32, "controller out"=w382:refnum<k24>)  [unwired: 6 in]
        n165 = call "GetAxisIndex.vi"("error in (no error)"=w380, "axis name"="Y", "controller in"=w382) -> ("error out"=w379:errorcluster, "axis index"=w373:i32, "controller out"=w381:refnum<k24>)  [unwired: 6 in]
        n166 = call "GetAxisIndex.vi"("error in (no error)"=w379, "axis name"="Z", "controller in"=w381) -> ("error out"=w357:errorcluster, "axis index"=w372:i32, "controller out"=w366:refnum<k24>)  [unwired: 6 in]
        n167 = Index Array(array=w375, index #1=w374, index #2=w373, index #3=w372) -> (element #1=w371:T6, element #2=w370:T6, element #3=w369:T6)
        n168 = Unbundle By Name(w369) -> ("Axis Status (str)"=w364:string, "Axis Status (bits).CommandValid"=w359:bool)
        n169 = Unbundle By Name(w370) -> ("Axis Status (str)"=w365:string, "Axis Status (bits).CommandValid"=w360:bool)
        n170 = Unbundle By Name(w371) -> ("Axis Status (str)"=w363:string, "Axis Status (bits).CommandValid"=w361:bool)
        n171 = case shown="True" w361 {
          frame False {
            n172 = property on="Enable X" class="Bool"("BoolText.Text"="ENABLE X") -> ()  [unwired: 2 in, 2 out]
          }
          frame True {
            n173 = property on="Enable X" class="Bool"("BoolText.Text"="DISABLE X") -> ()  [unwired: 2 in, 2 out]
          }
        }
        n174 = case shown="True" w360 {
          frame False {
            n175 = property on="Enable Y" class="Bool"("BoolText.Text"="ENABLE Y") -> ()  [unwired: 2 in, 2 out]
          }
          frame True {
            n176 = property on="Enable Y" class="Bool"("BoolText.Text"="DISABLE Y") -> ()  [unwired: 2 in, 2 out]
          }
        }
        n177 = case shown="True" w359 {
          frame False {
            n178 = property on="Enable Z" class="Bool"("BoolText.Text"="ENABLE Z") -> ()  [unwired: 2 in, 2 out]
          }
          frame True {
            n179 = property on="Enable Z" class="Bool"("BoolText.Text"="DISABLE Z") -> ()  [unwired: 2 in, 2 out]
          }
        }
        n180 = Bundle By Name(cluster=w368, "X"=w363, "X"=w361, "Y"=w365, "Y"=w360, "Z"=w364, "Z"=w359) -> (w367:T3)
      }
      frame "Idle" {
        n181 = event shown="[4] \"HOME U\": Value Change" {
          selector: _ -> [_ _ _ _ _ _ _ _ _ _ _]
          dyn-events: _ -> [_ _ _ _ _ _ _ _ _ _ _]
          timeout: 50 -> [_ _ _ _ _ _ _ _ _ _ _]
          tunnel: w402 -> [w425 w446 w452 w460 w472 w479 w496 w508 w512 w533 w550]
          tunnel: w403 -> [w426 w445 w454 w462 w470 w481 w497 w507 w511 w535 w556]
          tunnel: w401 -> [w406 w447 w455 w463 w468 w476 w498 w502 w514 w530 w552]
          tunnel: [SafeControl."Idle" SafeControl."Idle" SafeControl."Idle" SafeControl."Idle" SafeControl."Idle" SafeControl."Idle" SafeControl."Abort" SafeControl."Idle" SafeControl."Idle" SafeControl."Idle" SafeControl."Idle"] -> w400
          tunnel: [w425 w446 w452 w460 w471 w479 w496 w504 _ w533 w550] -> w399
          tunnel: [FALSE FALSE FALSE FALSE FALSE FALSE FALSE _ FALSE FALSE FALSE] -> w397
          tunnel: w396 -> [_ _ _ _ _ _ _ w506 _ _ _]
          tunnel: [w414 w447 w455 w463 w468 w476 w498 w502 w514 w530 w552] -> w395
          tunnel: [w410 w444 w453 w461 w469 w475 w497 w501 _ w529 w551] -> w394
          event Timeout {
            n182 = event-data() -> ()  [unwired: 1 in, 3 out]
            n183 = call "RetrieveDiagPacket.vi"("error in (no error)"=w426, "axisMask"=0, "Controller In"=w425) -> ("error out"=w439:errorcluster, "ControllerDiagPacket"=w440:T5, "Controller Out"=w438:refnum<k24>)  [unwired: 6 in]
            n184 = Unbundle(w440) -> ("Axes"=w430:T6[])  [unwired: 2 out]
            n185 = call "GetAxisIndex.vi"("error in (no error)"=w439, "axis name"="X", "controller in"=w438) -> ("error out"=w435:errorcluster, "axis index"=w429:i32, "controller out"=w437:refnum<k24>)  [unwired: 6 in]
            n186 = call "GetAxisIndex.vi"("error in (no error)"=w435, "axis name"="Y", "controller in"=w437) -> ("error out"=w434:errorcluster, "axis index"=w428:i32, "controller out"=w436:refnum<k24>)  [unwired: 6 in]
            n187 = call "GetAxisIndex.vi"("error in (no error)"=w434, "axis name"="Z", "controller in"=w436) -> ("error out"=w412:errorcluster, "axis index"=w427:i32, "controller out"=w411:refnum<k24>)  [unwired: 6 in]
            n188 = call "GetAxisIndex.vi"("error in (no error)"=w412, "axis name"="U", "controller in"=w411) -> ("error out"=w410:errorcluster, "axis index"=w408:i32)  [unwired: 6 in, 1 out]
            n189 = Index Array(array=w430, index #1=w429, index #2=w428, index #3=w427, index #4=w408) -> (element #1=w424:T6, element #2=w423:T6, element #3=w422:T6, element #4=w407:T6)
            n190 = Unbundle By Name(w422) -> ("Axis Status (str)"=w417:string, "Axis Status (bits).CommandValid"=w416:bool)
            n191 = Unbundle By Name(w423) -> ("Axis Status (str)"=w419:string, "Axis Status (bits).CommandValid"=w418:bool)
            n192 = Unbundle By Name(w407) -> ("Axis Status (str)"=w405:string, "Axis Status (bits).CommandValid"=w404:bool)
            n193 = Unbundle By Name(w424) -> ("Axis Status (str)"=w421:string, "Axis Status (bits).CommandValid"=w420:bool)
            n194 = Bundle By Name(cluster=w406, "X"=w421, "X"=w420, "Y"=w419, "Y"=w418, "Z"=w417, "Z"=w416, "U"=w405, "U"=w404) -> (w414:T3)
          }
          event "HOME X": Value Change {
            n195 = event-data() -> ()  [unwired: 1 in, 6 out]
            n196 = call "ExecuteCommand.vi"("error in (no error)"=w445, "taskId"=0, "Command Code"="HOME X", "controller in"=w446) -> ("error out"=w444:errorcluster)  [unwired: 5 in, 2 out]
          }
          event "HOME Y": Value Change {
            n197 = event-data() -> ()  [unwired: 1 in, 6 out]
            n198 = call "ExecuteCommand.vi"("error in (no error)"=w454, "taskId"=0, "Command Code"="HOME Y", "controller in"=w452) -> ("error out"=w453:errorcluster)  [unwired: 5 in, 2 out]
          }
          event "HOME Z": Value Change {
            n199 = event-data() -> ()  [unwired: 1 in, 6 out]
            n200 = call "ExecuteCommand.vi"("error in (no error)"=w462, "taskId"=0, "Command Code"="HOME Z", "controller in"=w460) -> ("error out"=w461:errorcluster)  [unwired: 5 in, 2 out]
          }
          event "HOME U": Value Change {
            n201 = event-data() -> ()  [unwired: 1 in, 6 out]
            n202 = call "ExecuteCommand.vi"("error in (no error)"=w470, "taskId"=0, "Command Code"="G90\nG0U2\nHOME U", "controller in"=w472) -> ("error out"=w469:errorcluster, "controller out"=w471:refnum<k24>)  [unwired: 5 in, 1 out]
          }
          event "Enable Y": Value Change {
            n203 = event-data() -> ()  [unwired: 1 in, 6 out]
            n204 = Unbundle By Name(w476) -> ("Y"=w478:bool)
            n205 = case shown="False" w478 {
              tunnel: w481 -> [w486 w492]
              tunnel: w479 -> [w485 w493]
              tunnel: [w482 w489] -> w475
              frame False {
                n206 = control-ref of="Enable Y"() -> (w484:refnum<vi>)
                n207 = call-poly "Enable.vi"("error in (no error)"=w486, "taskId"=0, "axis name"="Y", "controller in"=w485) -> ("error out"=w482:errorcluster)  [unwired: 6 in, 1 out]
                n208 = property class="Bool"(reference=w484, "BoolText.Text"="DISALBE Y") -> ()  [unwired: 1 in, 2 out]
              }
              frame True {
                n209 = control-ref of="Enable Y"() -> (w494:refnum<vi>)
                n210 = call-poly "Disable.vi"("error in (no error)"=w492, "taskId"=0, "axis name"="Y", "controller in"=w493) -> ("error out"=w489:errorcluster)  [unwired: 6 in, 1 out]
                n211 = property class="Bool"(reference=w494, "BoolText.Text"="ENABLE Y") -> ()  [unwired: 1 in, 2 out]
              }
            }
          }
          event "Exit": Value Change {
            n212 = event-data() -> ()  [unwired: 1 in, 6 out]
          }
          event "Excute": Value Change {
            n213 = event-data() -> ()  [unwired: 1 in, 6 out]
            n214 = call "ExecuteCommand.vi"("error in (no error)"=w507, "taskId"=0, "Command Code"=w506, "controller in"=w508) -> ("error out"=w501:errorcluster, "controller out"=w504:refnum<k24>)  [unwired: 5 in, 1 out]
          }
          event "Enable U": Value Change {
            n215 = event-data() -> ()  [unwired: 1 in, 6 out]
            n216 = Unbundle By Name(w514) -> ("U"=w513:bool)
            n217 = case shown="False" w513 {
              tunnel: w511 -> [w519 w526]
              tunnel: w512 -> [w518 w527]
              tunnel: [w516 w523] -> _
              frame False {
                n218 = control-ref of="Enable U"() -> (w515:refnum<vi>)
                n219 = call-poly "Enable.vi"("error in (no error)"=w519, "taskId"=0, "axis name"="U", "controller in"=w518) -> ("error out"=w516:errorcluster)  [unwired: 6 in, 1 out]
                n220 = property class="Bool"(reference=w515, "BoolText.Text"="DISALBE U") -> ()  [unwired: 1 in, 2 out]
              }
              frame True {
                n221 = control-ref of="Enable U"() -> (w522:refnum<vi>)
                n222 = call-poly "Disable.vi"("error in (no error)"=w526, "taskId"=0, "axis name"="U", "controller in"=w527) -> ("error out"=w523:errorcluster)  [unwired: 6 in, 1 out]
                n223 = property class="Bool"(reference=w522, "BoolText.Text"="ENABLE U") -> ()  [unwired: 1 in, 2 out]
              }
            }
          }
          event "Enable Z": Value Change {
            n224 = event-data() -> ()  [unwired: 1 in, 6 out]
            n225 = Unbundle By Name(w530) -> ("Z"=w532:bool)
            n226 = case shown="True" w532 {
              tunnel: w535 -> [w540 w546]
              tunnel: w533 -> [w539 w547]
              tunnel: [w536 w543] -> w529
              frame False {
                n227 = control-ref of="Enable Z"() -> (w538:refnum<vi>)
                n228 = property on="Property Node" class="Bool"(reference=w538, "BoolText.Text"="DISABLE Z") -> ()  [unwired: 1 in, 2 out]
                n229 = call-poly "Enable.vi"("error in (no error)"=w540, "taskId"=0, "axis name"="Z", "controller in"=w539) -> ("error out"=w536:errorcluster)  [unwired: 6 in, 1 out]
              }
              frame True {
                n230 = control-ref of="Enable Z"() -> (w548:refnum<vi>)
                n231 = call-poly "Disable.vi"("error in (no error)"=w546, "taskId"=0, "axis name"="Z", "controller in"=w547) -> ("error out"=w543:errorcluster)  [unwired: 6 in, 1 out]
                n232 = property on="Property Node" class="Bool"(reference=w548, "BoolText.Text"="ENABLE Z") -> ()  [unwired: 1 in, 2 out]
              }
            }
          }
          event "Enable X": Value Change {
            n233 = event-data() -> ()  [unwired: 1 in, 6 out]
            n234 = Unbundle By Name(w552) -> ("X"=w555:bool)
            n235 = case shown="False" w555 {
              tunnel: w550 -> [w560 w568]
              tunnel: w556 -> [w559 w567]
              tunnel: [w557 w563] -> w551
              frame False {
                n236 = property on="Enable X" class="Bool"("BoolText.Text"="DISABLE X") -> ()  [unwired: 2 in, 2 out]
                n237 = call-poly "Enable.vi"("error in (no error)"=w559, "taskId"=0, "axis name"="X", "controller in"=w560) -> ("error out"=w557:errorcluster)  [unwired: 6 in, 1 out]
              }
              frame True {
                n238 = control-ref of="Enable X"() -> (w564:refnum<vi>)
                n239 = property on="Property Node" class="Bool"(reference=w564, "BoolText.Text"="ENABLE X") -> ()  [unwired: 1 in, 2 out]
                n240 = call-poly "Disable.vi"("error in (no error)"=w567, "taskId"=0, "axis name"="X", "controller in"=w568) -> ("error out"=w563:errorcluster)  [unwired: 6 in, 1 out]
              }
            }
          }
        }
      }
      frame "Abort" {
      }
    }
    "Boolean" <- w336
    n241 = Unbundle By Name(w343) -> ("U"=→"U":bool, "X"=→"X":bool, "Y"=→"Y":bool, "Z"=→"Z":bool, "X"=→"X":string, "Y"=→"Y":string, "Z"=→"Z":string, "U"=→"U":string)
  }
  n242 = Merge Errors(w1, w4, w7) -> (w6:errorcluster)
  n243 = call "Disconnect.vi"("error in (no error)"=w6, "controller"=w2) -> ("error out"=w5:errorcluster)  [unwired: 9 in]
  n244 = call <vilib>:"Simple Error Handler.vi"("error in (no error)"=w5) -> ()  [unwired: 4 in, 5 out]
